vi "toEnum.vi"(11 "Instruction":bool) -> (3 "Enable/Disable?":u8)   [LabVIEW 2018]
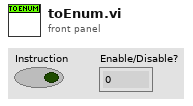
[diagram p1: front panel]
types:
  T1 = enum8{"Enabled", "Disabled", "Disabled and Grayed Out"}
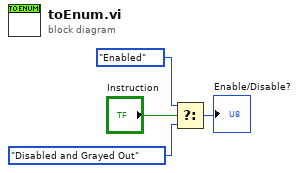
[diagram p0: block diagram]
diagram:
  n1 = Select(t=T1."Enabled" ("Disabled"), s="Instruction", f=T1."Disabled and Grayed Out" ("Disabled")) -> (s? t:f=→"Enable/Disable?":T1)
